vi "PointConvert.vi"(8 "RealWorldY":dbl format="%#_13g", 9 "RealWorldX":dbl format="%#_13g", 10 "RealWorldXY":cluster{"X":dbl, "Y":dbl}[][](array[cluster]), 11 "DeltaXY":cluster{dbl, dbl}[][](array[cluster])) -> (0 "DeltaY":dbl format="%#_13g", 1 "DeltaX":dbl format="%#_13g", 3 "100%?":bool)   [LabVIEW 2019]
panel:
  out "element 2":dbl
  out "element":dbl
  out "ansX":dbl
  out "ansY":dbl
  out "element 12":cluster{"X":dbl, "Y":dbl}
  out "element 11":cluster{"X":dbl, "Y":dbl}
  out "element 10":cluster{"X":dbl, "Y":dbl}
  out "element 9":cluster{"X":dbl, "Y":dbl}
  out "element 8":cluster{"X":dbl, "Y":dbl}
  out "element 7":cluster{"X":dbl, "Y":dbl}
  out "element 6":cluster{"X":dbl, "Y":dbl}
  out "element 5":cluster{"X":dbl, "Y":dbl}
  out "Array 2":dbl[][](array[numeric])
  out "Numeric":dbl
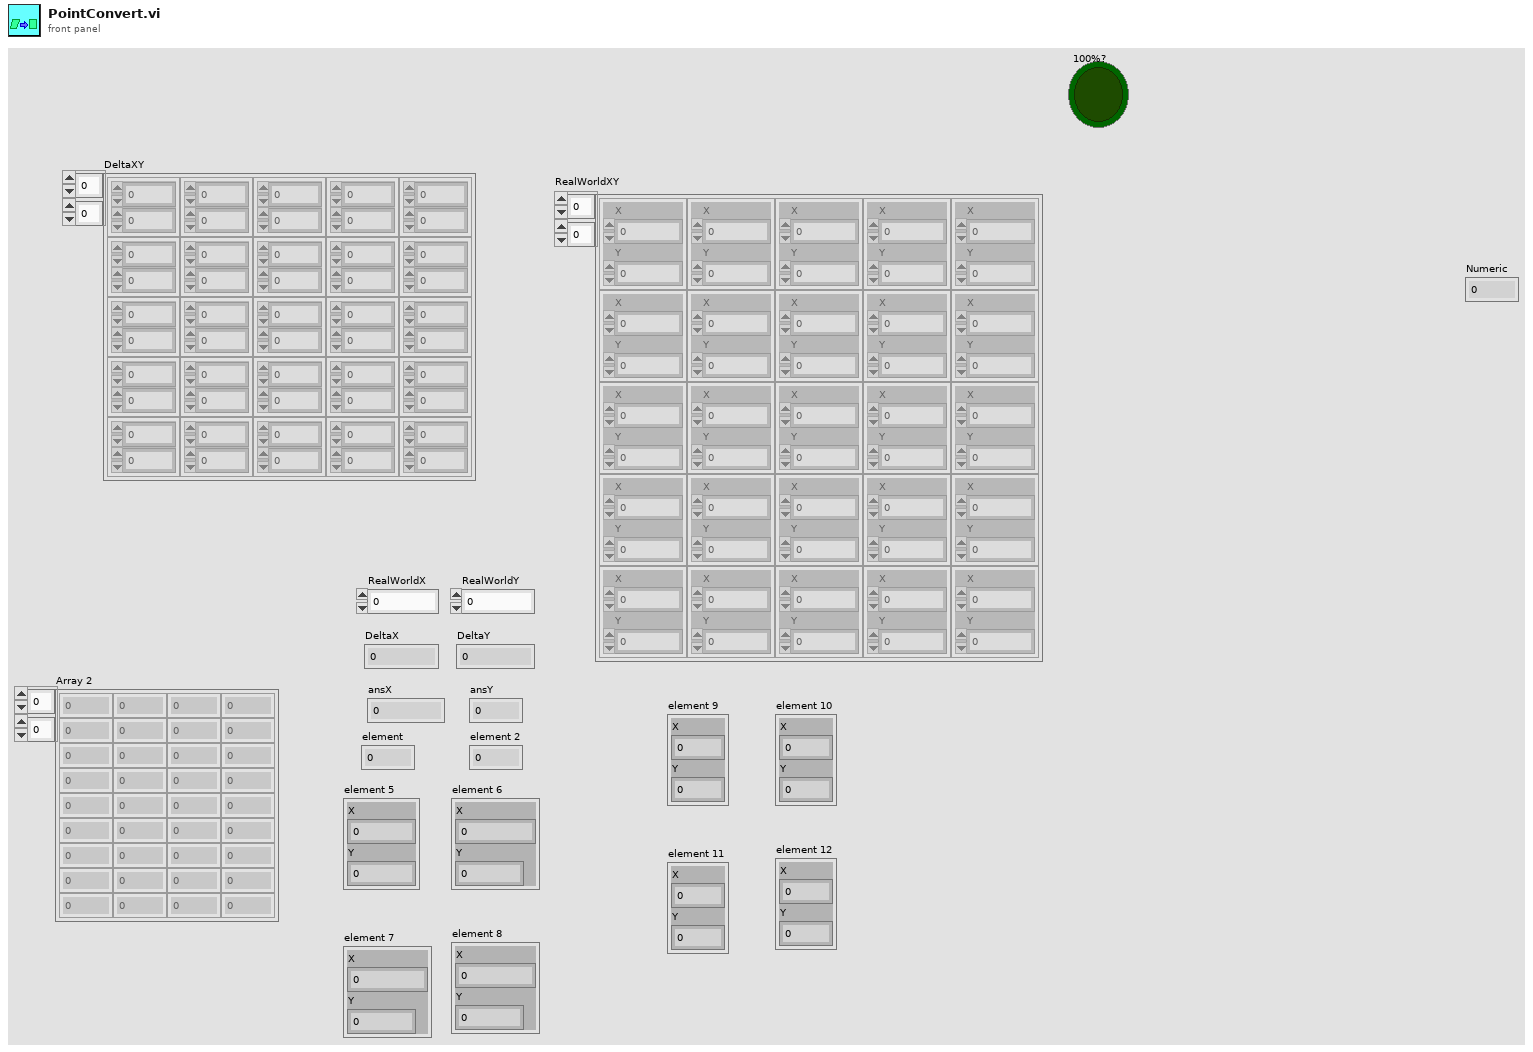
[diagram p1: front panel]
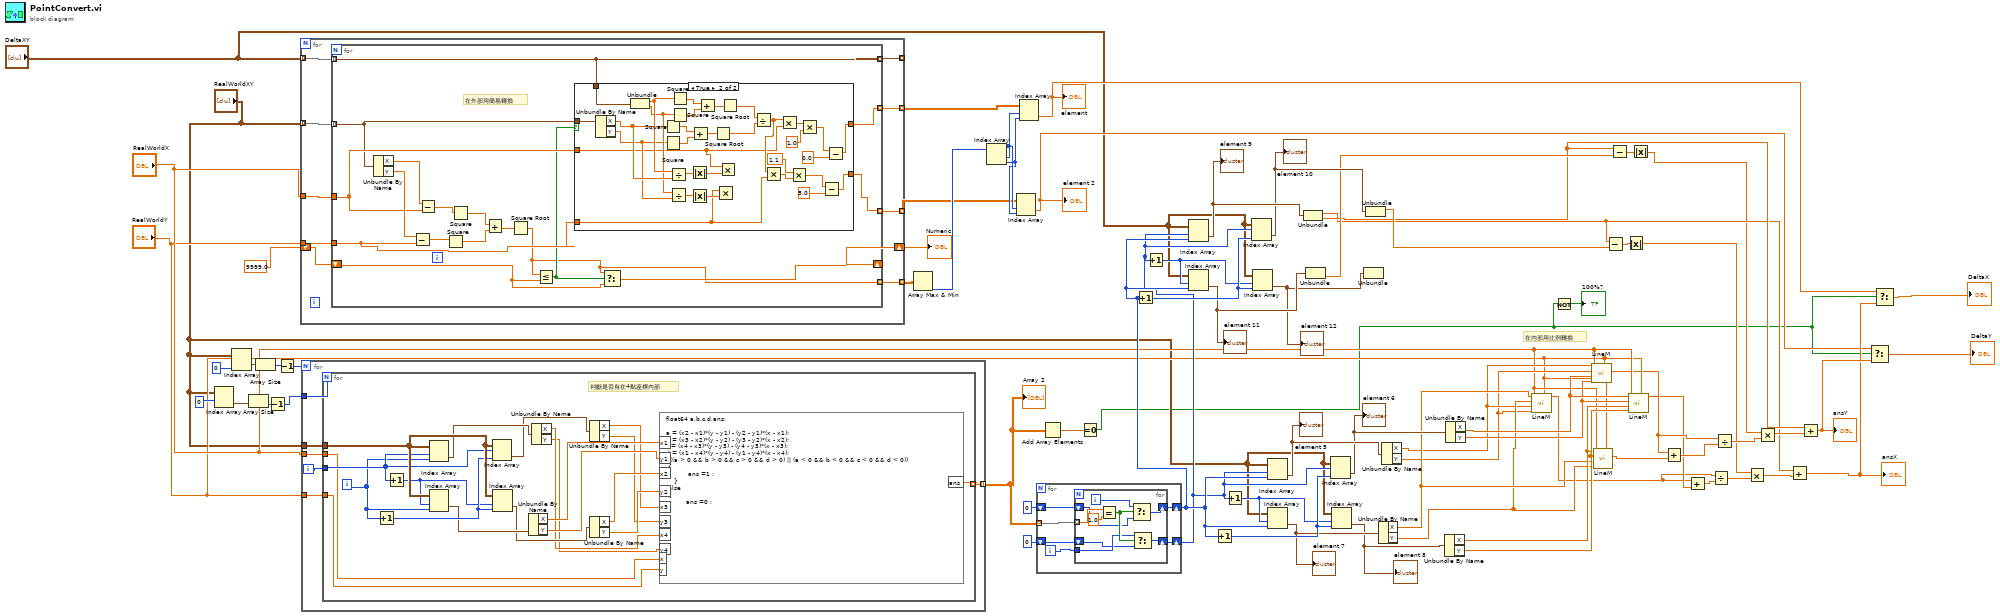
[diagram p0: block diagram]
diagram:
  # "在內部用比例轉換"
  n1 = Index Array(array="RealWorldXY", index (row)=0 ("index (col)")) -> (element=w61:cluster{"X":dbl, "Y":dbl}[])  [unwired: 1 in]
  n2 = Index Array(array="RealWorldXY", index (col)=0 ("index (row)")) -> (element=w66:cluster{"X":dbl, "Y":dbl}[])  [unwired: 1 in]
  n3 = Array Size(array=w61) -> (size(s)=w63:i32)
  n4 = Array Size(array=w66) -> (size(s)=w65:i32)
  n5 = Decrement(x=w63) -> (x-1=w62:i32)
  n6 = Decrement(x=w65) -> (x-1=w64:i32)
  n7 = for {
    tunnel: "RealWorldXY" -> [w75] mode=indexing
    tunnel: "RealWorldX" -> [w82]
    tunnel: "RealWorldY" -> [w81]
    tunnel: [w80] -> _ mode=indexing
    tunnel: "DeltaXY" -> [w79] mode=indexing
    tunnel: [w78] -> w72 mode=indexing
    tunnel: [w77] -> w71 mode=indexing
    tunnel: [w76] -> w67 mode=indexing
    shift-right: [w74] -> w4
    shift-left: 9999.0 -> [w73]
    n8 = for {
      tunnel: w75 -> [w83] mode=indexing
      tunnel: w82 -> [w91]
      tunnel: w81 -> [w90]
      tunnel: [w92] -> w80 mode=indexing
      tunnel: w79 -> [w92] mode=indexing
      shift-right: [w88] -> w74
      shift-left: w73 -> [w87]
      tunnel: [w86] -> w78 mode=indexing
      tunnel: [w85] -> w77 mode=indexing
      tunnel: [w84] -> w76 mode=indexing
      # "在外部用簡易轉換"
      n9 = Unbundle By Name(w83) -> ("X"=w99:dbl, "Y"=w98:dbl)
      n10 = Subtract(x=w98, y=w90) -> (x-y=w96:dbl)
      n11 = Subtract(x=w99, y=w91) -> (x-y=w97:dbl)
      n12 = Square(x=w96) -> (x^2=w94:dbl)
      n13 = Square(x=w97) -> (x^2=w95:dbl)
      n14 = Add(x=w95, y=w94) -> (x+y=w93:dbl)
      n15 = Square Root(x=w93) -> (sqrt(x)=w86:dbl)
      n16 = Less Or Equal?(x=w86, y=w87) -> (x <= y?=w89:bool)
      n17 = case shown="True" w89 {
        tunnel: w92 -> [_ w131]
        tunnel: w83 -> [_ w132]
        tunnel: w91 -> [w101 w111]
        tunnel: w90 -> [w100 w110]
        tunnel: [w101 w105] -> w85
        tunnel: [w100 w102] -> w84
        frame False {
        }
        frame True {
          n18 = Unbundle By Name(w132) -> ("X"=w118:dbl, "Y"=w116:dbl)
          n19 = Unbundle(w131) -> (w119:dbl, w117:dbl)
          n20 = Square(x=w118) -> (x^2=w127:dbl)
          n21 = Square(x=w116) -> (x^2=w126:dbl)
          n22 = Divide(x=w119, y=w118) -> (x/y=w115:dbl)
          n23 = Divide(x=w117, y=w116) -> (x/y=w114:dbl)
          n24 = Square(x=w119) -> (x^2=w128:dbl)
          n25 = Square(x=w117) -> (x^2=w129:dbl)
          n26 = Absolute Value(x=w115) -> (abs(x)=w112:dbl)
          n27 = Absolute Value(x=w114) -> (abs(x)=w113:dbl)
          n28 = Add(x=w127, y=w126) -> (x+y=w125:dbl)
          n29 = Add(x=w128, y=w129) -> (x+y=w130:dbl)
          n30 = Square Root(x=w125) -> (sqrt(x)=w123:dbl)
          n31 = Multiply(x=w110, y=w113) -> ()  [unwired: 1 out]
          n32 = Multiply(x=w111, y=w112) -> ()  [unwired: 1 out]
          n33 = Square Root(x=w130) -> (sqrt(x)=w124:dbl)
          n34 = Divide(x=w124, y=w123) -> (x/y=w121:dbl)
          n35 = Multiply(x=w121, y=w110) -> (x*y=w108:dbl)
          n36 = Multiply(x=w121, y=w111) -> (x*y=w109:dbl)
          n37 = Multiply(x=1.1, y=w108) -> (x*y=w103:dbl)
          n38 = Multiply(x=w109, y=1.0) -> (x*y=w107:dbl)
          n39 = Subtract(x=w103, y=5.0) -> (x-y=w102:dbl)
          n40 = Subtract(x=w107, y=0.0) -> (x-y=w105:dbl)
        }
      }
      n41 = Select(t=w86, s=w89, f=w87) -> (s? t:f=w88:dbl)
    }
  }
  "Numeric" <- w4
  n42 = for {
    N: w64 -> [_]
    tunnel: "RealWorldX" -> [w138]
    tunnel: "RealWorldY" -> [w137]
    tunnel: "RealWorldXY" -> [w135]
    tunnel: w62 -> [w134]
    tunnel: [w133] -> w57 mode=indexing
    i -> [w136]
    n43 = for {
      N: w134 -> [_]
      tunnel: w138 -> [w141]
      tunnel: w137 -> [w140]
      tunnel: w136 -> [w157]
      tunnel: w135 -> [w158]
      tunnel: [w139] -> w133 mode=indexing
      i -> [w154]
      # "判斷是否有在4點座標內部"
      n44 = Increment(x=w154) -> (x+1=w156:i32)
      n45 = Increment(x=w157) -> (x+1=w155:i32)
      n46 = Index Array(array=w158, index (row)=w157, index (col)=w154) -> (element=w153:cluster{"X":dbl, "Y":dbl})
      n47 = Index Array(array=w158, index (row)=w155, index (col)=w154) -> (element=w151:cluster{"X":dbl, "Y":dbl})
      n48 = Index Array(array=w158, index (row)=w157, index (col)=w156) -> (element=w152:cluster{"X":dbl, "Y":dbl})
      n49 = Index Array(array=w158, index (row)=w155, index (col)=w156) -> (element=w150:cluster{"X":dbl, "Y":dbl})
      n50 = Unbundle By Name(w151) -> ("X"=w149:dbl, "Y"=w148:dbl)
      n51 = Unbundle By Name(w153) -> ("X"=w143:dbl, "Y"=w142:dbl)
      n52 = Unbundle By Name(w152) -> ("X"=w145:dbl, "Y"=w144:dbl)
      n53 = Unbundle By Name(w150) -> ("X"=w147:dbl, "Y"=w146:dbl)
      n54 = formula code="float64 a,b,c,d,ans;\n\na = (x2 - x1)*(y - y1) - (y2 - y1)*(x - x1);  \nb = (x3 - x2)*(y - y2) - (y3 - y2)*(x - x2);  \nc = (x4 - x3)*(y - y3) - (y4 - y3)*(x - x3);  \nd = (x1 - x4)*(y - y4) - (y1 - y4)*(x - x4);  \nif((a > 0 && b > 0 && c > 0 && d > 0) || (a < 0 && b < 0 && c < 0 && d < 0)) \n\t{  \n           ans =1 ;  \n    }  \n\telse\n\t{\n\t\t        ans =0 ;\n\t}"("x1"=w149, "y1"=w148, "x2"=w147, "y2"=w146, "x3"=w145, "y3"=w144, "x4"=w143, "y4"=w142, "x"=w141, "y"=w140) -> ("ans"=w139:dbl)
    }
  }
  "Array 2" <- w57
  n55 = Array Max & Min(array=w72) -> (min index (indices)=w70:i32[])  [unwired: 3 out]
  n56 = Index Array(array=w70) -> (element #1=w69:i32, element #2=w68:i32)  [unwired: 2 in]
  n57 = Index Array(array=w67, index (row)=w69, index (col)=w68) -> (element=w9:dbl)
  "element 2" <- w9
  n58 = Index Array(array=w71, index (row)=w69, index (col)=w68) -> (element=w10:dbl)
  "element" <- w10
  n59 = for {
    tunnel: w57 -> [w164] mode=indexing
    shift-right: [w162] -> w42
    shift-left: 0 -> [w161]
    shift-right: [w160] -> w41
    shift-left: 0 -> [w159]
    i -> [w163]
    n60 = for {
      tunnel: w164 -> [w173] mode=indexing
      tunnel: w163 -> [w168]
      shift-right: [w169] -> w162
      shift-left: w161 -> [w165]
      shift-right: [w167] -> w160
      shift-left: w159 -> [w166]
      i -> [w170]
      n61 = Equal?(x=w173, y=1.0) -> (x = y?=w171:bool)
      n62 = Select(t=w170, s=w171, f=w165) -> (s? t:f=w169:i32)
      n63 = Select(t=w168, s=w171, f=w166) -> (s? t:f=w167:i32)
    }
  }
  n64 = Add Array Elements(numeric array=w57) -> (sum=w58:dbl)
  n65 = Equal To 0?(x=w58) -> (x = 0?=w2:bool)
  n66 = Increment(x=w42) -> (x+1=w48:i32)
  n67 = Increment(x=w41) -> (x+1=w47:i32)
  n68 = Index Array(array="DeltaXY", index (row)=w41, index (col)=w42) -> (element=w46:cluster{dbl, dbl})
  "element 9" <- w46
  n69 = Index Array(array="DeltaXY", index (row)=w47, index (col)=w42) -> (element=w44:cluster{dbl, dbl})
  "element 11" <- w44
  n70 = Increment(x=w42) -> (x+1=w54:i32)
  n71 = Increment(x=w41) -> (x+1=w53:i32)
  n72 = Index Array(array="DeltaXY", index (row)=w41, index (col)=w48) -> (element=w45:cluster{dbl, dbl})
  "element 10" <- w45
  n73 = Index Array(array="DeltaXY", index (row)=w47, index (col)=w48) -> (element=w43:cluster{dbl, dbl})
  "element 12" <- w43
  n74 = Index Array(array="RealWorldXY", index (row)=w41, index (col)=w42) -> (element=w52:cluster{"X":dbl, "Y":dbl})
  "element 5" <- w52
  n75 = Index Array(array="RealWorldXY", index (row)=w53, index (col)=w42) -> (element=w50:cluster{"X":dbl, "Y":dbl})
  "element 7" <- w50
  n76 = Unbundle(w46) -> (w17:dbl, w20:dbl)
  n77 = Unbundle(w44) -> (w24:dbl)  [unwired: 1 out]
  n78 = Index Array(array="RealWorldXY", index (row)=w41, index (col)=w54) -> (element=w51:cluster{"X":dbl, "Y":dbl})
  "element 6" <- w51
  n79 = Index Array(array="RealWorldXY", index (row)=w53, index (col)=w54) -> (element=w49:cluster{"X":dbl, "Y":dbl})
  "element 8" <- w49
  n80 = Unbundle(w43) -> ()  [unwired: 2 out]
  n81 = Unbundle(w45) -> (w23:dbl)  [unwired: 1 out]
  n82 = Unbundle By Name(w50) -> ("X"=w36:dbl, "Y"=w35:dbl)
  n83 = Unbundle By Name(w52) -> ("X"=w34:dbl, "Y"=w33:dbl)
  n84 = Unbundle By Name(w49) -> ("X"=w37:dbl, "Y"=w38:dbl)
  n85 = Unbundle By Name(w51) -> ("X"=w40:dbl, "Y"=w39:dbl)
  n86 = call "LineM.vi"("Yin"="RealWorldY", "Xin"="RealWorldX", "Y2"=w33, "X2"=w34, "Y1"=w35, "X1"=w36) -> ("Xdistance"=w25:dbl)  [unwired: 1 in, 4 out]
  n87 = Not(x=w2) -> (.not. x?=→"100%?":bool)
  n88 = call "LineM.vi"("Yin"="RealWorldY", "Xin"="RealWorldX", "Y2"=w39, "X2"=w40, "Y1"=w33, "X1"=w34) -> ("Ydistance"=w29:dbl)  [unwired: 1 in, 4 out]
  n89 = call "LineM.vi"("Yin"="RealWorldY", "Xin"="RealWorldX", "Y2"=w35, "X2"=w36, "Y1"=w38, "X1"=w37) -> ("Ydistance"=w30:dbl)  [unwired: 1 in, 4 out]
  n90 = Subtract(x=w17, y=w23) -> (x-y=w16:dbl)
  n91 = Subtract(x=w20, y=w24) -> (x-y=w14:dbl)
  n92 = Absolute Value(x=w16) -> (abs(x)=w15:dbl)
  n93 = call "LineM.vi"("Yin"="RealWorldY", "Xin"="RealWorldX", "Y2"=w38, "X2"=w37, "Y1"=w39, "X1"=w40) -> ("Xdistance"=w27:dbl)  [unwired: 1 in, 4 out]
  n94 = Absolute Value(x=w14) -> (abs(x)=w13:dbl)
  n95 = Add(x=w29, y=w30) -> (x+y=w28:dbl)
  n96 = Add(x=w25, y=w27) -> (x+y=w26:dbl)
  n97 = Divide(x=w25, y=w26) -> (x/y=w18:dbl)
  n98 = Divide(x=w29, y=w28) -> (x/y=w22:dbl)
  n99 = Multiply(x=w15, y=w18) -> (x*y=w19:dbl)
  n100 = Multiply(x=w13, y=w22) -> (x*y=w21:dbl)
  n101 = Add(x=w17, y=w19) -> (x+y=w11:dbl)
  "ansX" <- w11
  n102 = Add(x=w20, y=w21) -> (x+y=w12:dbl)
  "ansY" <- w12
  n103 = Select(t=w9, s=w2, f=w12) -> (s? t:f=→"DeltaY":dbl)
  n104 = Select(t=w10, s=w2, f=w11) -> (s? t:f=→"DeltaX":dbl)
